vi "Roughness Averager Create.vi"(8 "error in (no error)":errorcluster, 9 "Full? (T)":bool=TRUE, 10 "SubSampling Interval (10)":i32=10, 11 "Roughness Averager in":refnum<class "Roughness Averager.lvclass">) -> (0 "error out":errorcluster, 3 "Roughness Averager out":refnum<class "Roughness Averager.lvclass">)   [LabVIEW 2018, in "Roughness Averager.lvclass"]
uses:
  Roughness Averager.lvclass
  Roughness Averager.lvclass/Roughness Averager.ctl
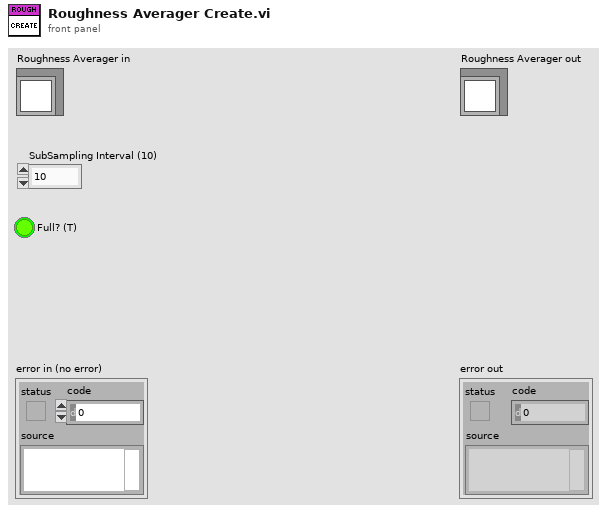
[diagram p1: front panel]
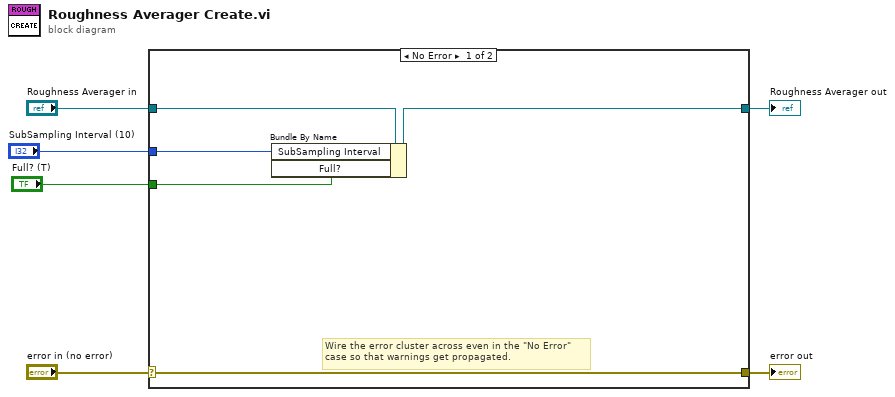
[diagram p0: block diagram]
diagram:
  n1 = case shown="No Error" "error in (no error)" {
    selector: "error in (no error)" -> [w11 w13]
    tunnel: [w11 w13] -> w5
    tunnel: [w8 w12] -> w3
    tunnel: "Roughness Averager in" -> [w10 w12]
    tunnel: "SubSampling Interval (10)" -> [w9 _]
    tunnel: "Full? (T)" -> [w7 _]
    frame No Error {
      # "Wire the error cluster across even in the \"No Error\"\ncase so that warnings get propagated."
      n2 = Bundle By Name(cluster=w10, "SubSampling Interval"=w9, "Full?"=w7) -> (w8:refnum<class "Roughness Averager.lvclass">)
    }
    frame Error {
    }
  }
  "error out" <- w5
  "Roughness Averager out" <- w3
